vi "03记录拆表格.vi"(1 "03类（被收）":string[](array[string])) -> (15 "拆分显示（主页）":string[][](array[string]))   [LabVIEW 2019]
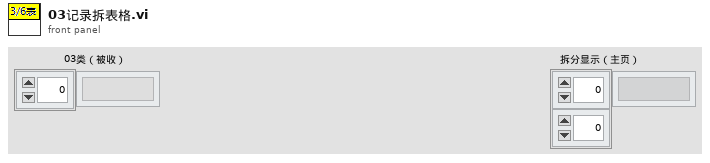
[diagram p1: front panel]
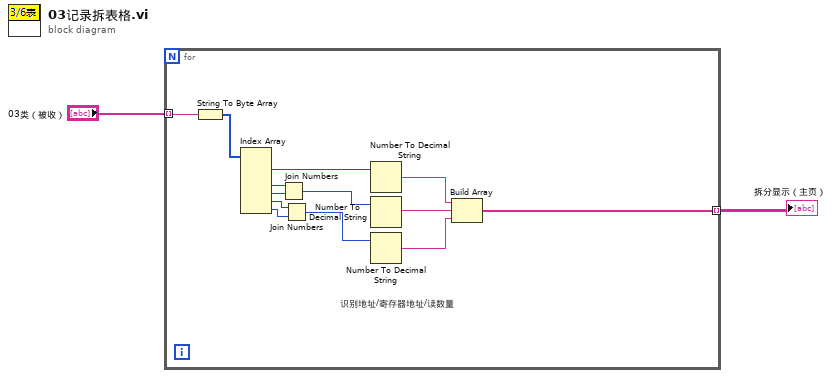
[diagram p0: block diagram]
diagram:
  n1 = for {
    tunnel: "03类（被收）" -> [w15] mode=indexing
    tunnel: [w3] -> w1 mode=indexing
    # "识别地址/寄存器地址/读数量"
    n2 = String To Byte Array(string=w15) -> (unsigned byte array=w7:u8[])
    n3 = Index Array(array=w7) -> (element #1=w12:u8, element #3=w8:u8, element #4=w9:u8, element #5=w10:u8, element #6=w11:u8)  [unwired: 6 in, 1 out]
    n4 = Join Numbers(hi=w8, lo=w9) -> ((hi.lo)=w13:u16)
    n5 = Join Numbers(hi=w10, lo=w11) -> ((hi.lo)=w14:u16)
    n6 = Number To Decimal String(number=w12) -> (decimal integer string=w6:string)  [unwired: 1 in]
    n7 = Number To Decimal String(number=w13) -> (decimal integer string=w5:string)  [unwired: 1 in]
    n8 = Number To Decimal String(number=w14) -> (decimal integer string=w4:string)  [unwired: 1 in]
    n9 = Build Array(w6, w5, w4) -> (w3:string[])
  }
  "拆分显示（主页）" <- w1
